vi "Litremeter func glob.vi"(5 "Action":enum16{"Get", "Set"}(ring), 6 "Offset Litres in":dbl, 7 "Litres / pulse in":dbl=1.0, 8 "Pulse count in":u32, 9 "Counter task in":refnum<k21>) -> (0 "Offset Litres out":dbl, 1 "Litres / pulse out":dbl=1.0, 2 "Pulse count out":u32, 3 "Counter task out":refnum<k21>, 4 "Total Litres (calc)":dbl)   [LabVIEW 2011]
panel:
  # "by Paul Nathan, 01/03/2012"
  # "Revisions:\nDate       Desc.      Auth.\nx               x               x"
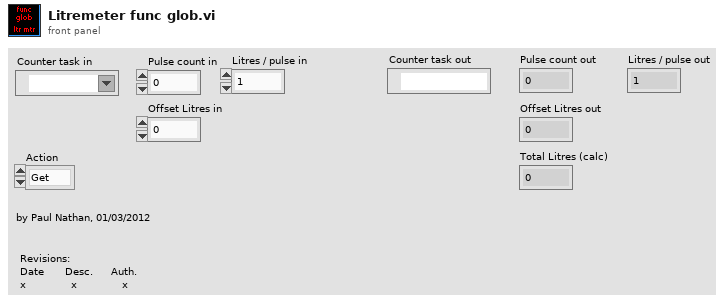
[diagram p1: front panel]
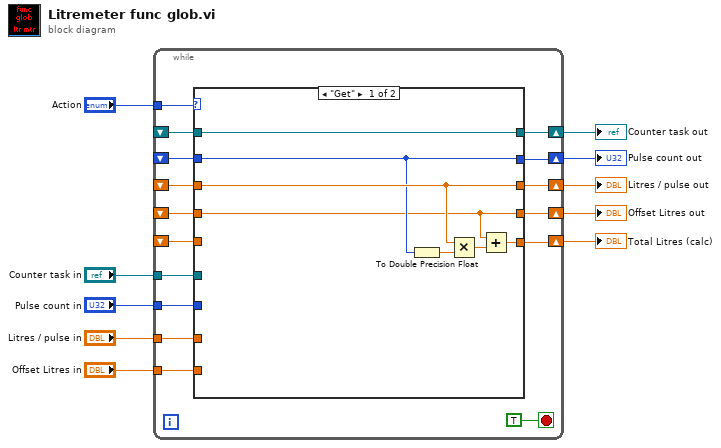
[diagram p0: block diagram]
diagram:
  n1 = while {
    tunnel: "Action" -> [w25]
    shift-right: [w23] -> w6
    shift-left: _ -> [w24]
    shift-right: [w22] -> w5
    shift-left: _ -> [w20]
    shift-right: [w21] -> w4
    shift-left: _ -> [w19]
    tunnel: "Counter task in" -> [w18]
    tunnel: "Pulse count in" -> [w17]
    tunnel: "Litres / pulse in" -> [w16]
    shift-right: [w13] -> w2
    shift-left: _ -> [w14]
    tunnel: "Offset Litres in" -> [w15]
    shift-right: [w12] -> w1
    shift-left: _ -> [w11]
    stop <- TRUE stop-if-true
    n2 = case shown="\"Get\"" w25 {
      tunnel: w24 -> [w33 _]
      tunnel: [w33 w38] -> w23
      tunnel: [w30 w37] -> w22
      tunnel: [w32 w36] -> w21
      tunnel: w20 -> [w30 _]
      tunnel: w19 -> [w32 _]
      tunnel: w18 -> [_ w38]
      tunnel: w17 -> [_ w37]
      tunnel: w16 -> [_ w36]
      tunnel: w15 -> [_ w35]
      tunnel: w14 -> [w27 _]
      tunnel: [w27 w35] -> w13
      tunnel: [w29 w34] -> w12
      tunnel: w11 -> [_ w34]
      frame "Get" {
        n3 = To Double Precision Float(number=w30) -> (double precision float=w31:dbl)
        n4 = Multiply(x=w32, y=w31) -> (x*y=w28:dbl)
        n5 = Add(x=w27, y=w28) -> (x+y=w29:dbl)
      }
      frame "Set" {
      }
    }
  }
  "Counter task out" <- w6
  "Pulse count out" <- w5
  "Litres / pulse out" <- w4
  "Offset Litres out" <- w2
  "Total Litres (calc)" <- w1
